vi "AlliGator Build Background Dataset Information String.vi"(8 "error in (no error)":errorcluster, 11 "Bkgd Subtraction":bool) -> (0 "error out":errorcluster, 3 "Background Dataset Description":string)   [LabVIEW 2021, in "AlliGator Files.lvlib"]
doc: "Builds background dataset information string."
uses:
  AlliGator Files.lvlib
  Globals, Variables, Constants/AlliGator Variables List.ctl
  Variant/Variant to Data/Variant to Path.vi
  Variant/Variant to Data/Variant to Boolean.vi
  Variant/Variant to Data/Variant to U32.vi
  Variant/Variant to Data/Variant to DBL.vi
  Variant/Variant to Data/Variant to String.vi
  Globals, Variables, Constants/AlliGator Globals, Variables & Constants.lvlib
  Variant/Variant to Data/Variant to Data.lvlib
panel:
  # "see the AlliGator License on the block diagram (Ctrl+E or Window:Show Block Diagram)"
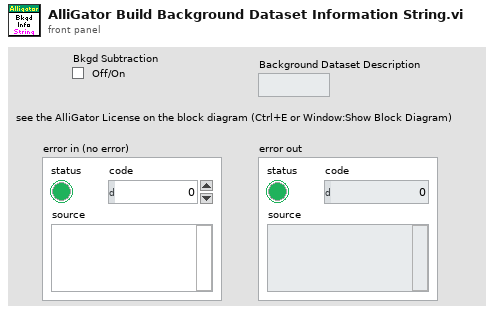
[diagram p1: front panel]
types:
  T1 = typedef "AlliGator Globals, Variables & Constants.lvlib/AlliGator Variables List.ctl" = enum16{"---- GUI ----", "GUI:Initialization Status", "GUI:State Indicators Refnum", "GUI:Original AlliGator Menu Items", "GUI:Current Action Loop State", "GUI:Script in progress", "GUI:Playback", "GUI:Loop Playback", "GUI:Search ROI Used", "GUI:Search ROI", "Decay Graph Max Legend Size", "Intensity Graph Max Legend Size", "Decay Statistics Graph Max Legend Size", "Phasor Graph Max Legend Size", "Phasor Ratio Graph Max Legend Size", "Lifetime Graph Max Legend Size", "---- Files ----", "Files:Export Dataset Frames as Individual Files", "Files:Show Batch Export Help Balloons", "Files:Frames in Dataset", "Files:ptu File Frame Start Indices", "Files:Current Frame in Dataset", "Files:Current Frame Timestamp", "Files:Dataset Loaded", "Files:Dataset Metadata", "Files:Dataset Channel", "Files:Dataset Data Description", "Files:Background Dataset Metadata", "Files:Background Dataset Channel", "Files:Background Dataset Data Description", "Files:Background File Subtraction", "Files:Background File Path", "Files:Background File Pile-up Correction", "Files:Background File Pixel Well Capacity", "Files:Background File Scaling Factor", "Files:Current Dataset Load Settings", "Files:Dataset Path", "Files:ICCD-specific Information", "Files:Macrotime Gate Separation", "------ Python Plugins ------", "Python Plugins:Information", "Python Plugins:Python Session", "Python Plugins:Valid Python Session?", "---- Source Image ----", "Source Image:ROIs", "Source Image:Current ROI", "Source Image:ROI Event Refnum", "X_Source Image Display Range", "X_Source Image Palette Information", "X_Type of Displayed Image", "X_Time Gate Slider", "Source Image:Palette List", "Source Image:Scale", "Source Image:ROI Overlay Color", "Source Image:Overlay to Erase", "Source Image:Is Displayed Image Accumulated", "Source Image:White Light Image Modified", "Source Image:Mask Image Modified", "---- Image Profile Window ----", "Image Profile:Window Event Refnum", "Image Profile:IntensityType", "Image Profile:Intensity Average Type", "Image Profile:Intensity-weighted SDV", "Image Profile:Box Profile Type", "Image Profile:Window Open", "Image Profile:Plotted Fit Parameter", "------ Phasor Graph -------", "Phasor Graph:Show Line", "---- Phasor Plot ---", "Phasor Plot:Parameters Changed", "Phasor Plot:FLI Dataset Modified since last Calculation", "Phasor Harmonics Data", "Selected Phasor Harmonics", "Phasor Harmonic Manager Event Refnum", "Phasor Plot:ROIs", "Phasor Plot:Current ROI", "Phasor Plot:ROI Event Refnum", "Phasor Plot:Image Reference Points", "Phasor Plot:Computed", "Phasor Plot:Palette Information", "Phasor Plot:Palette List", "Phasor Plot:Phasor Ratio Palette Information", "Phasor Plot:Phasor Ratio Palette List", "Phasor Plot:Image Scale", "Phasor Plot:Image Overlay to Erase", "Phasor Plot:Image Elements to Update", "Phasor Plot:Current Calculation Parameters", "Phasor Plot:Current Calibration Options", "Phasor Plot:Reset Cumulated Phasor Plot", "Phasor Plot:Reference 1", "Phasor Plot:Lifetime Reference 1", "Phasor Plot:Reference 1 Frequency", "Phasor Plot:Reference 2", "Phasor Plot:Lifetime Reference 2", "Phasor Plot:Reference 2 Frequency", "---- Decay Analysis ----", "Number of Selected Decays to Fit", "LS Fit Results", "LAR Fit Results", "BS Fit Results", "Last Decay Max - Min", "Best Fit Parameters", "Best Fit Parameter Names", "Actual Size X", "Actual Size Y", "Binning X", "Binning Y", "Actual # Gates", "Dataset Number", "Gates to...", "Gates Skipped", "Gates to keep", "Gate Step", "Gate Separation", "Reversed Gates", "Pile-up Correction", "Pixel Well Capacity", "Background Subtracted", "Background Subtraction Method", "Background Definition Range", "Background File (deprecated)", "Number of Dataset Accumulated", "Array of Accumulated Dataset Paths", "Do Averaged Datasets", "Destination File Path", "Process Plot Target", "Use 1/D as Phasor Frequency", "---- Decay Fit Parameter Map -----", "Decay Fit Parameter Map:Palette Information", "Decay Fit Parameter Map:Palette List", "---- Parameter Map ----", "Parameter Map:Palette Information", "Parameter Map:Palette List", "------- Local Decay Window ---------", "Local Decay Graph Window:Event Refnum", "Local Decay Graph Window:Use normalized IRF for convolution", "----- Miscellaneous ----", "Misc:Skippable Dialog Windows Status"}
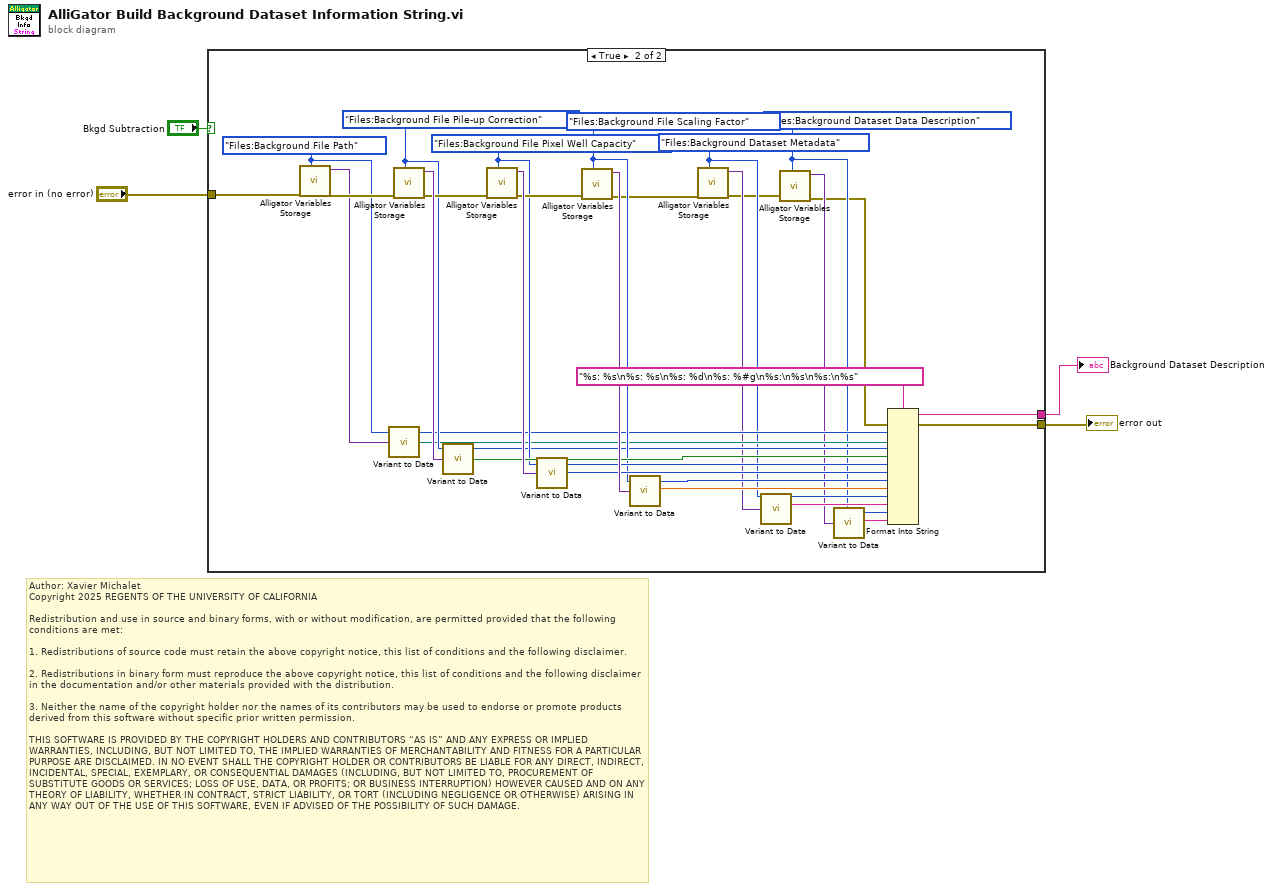
[diagram p0: block diagram]
diagram:
  # "Author: Xavier Michalet\nCopyright 2025 REGENTS OF THE UNIVERSITY OF CALIFORNIA\n\nRedistribution and use in source and binary forms, with or without modification, are permitted provided that the following conditions are met:\n\n1. Redistributions of source code must retain the above copyright notice, this list of conditions and the following disclaimer.\n\n2. Redistributions in binary form must reproduce the above copyright notice, this list of conditions and the following disclaimer in the documentation and/or other materials provided with the distribution.\n\n3. Neither the name of the copyright holder nor the names of its contributors may be used to endorse or promote products derived from this software without specific prior written permission.\n\nTHIS SOFTWARE IS PROVIDED BY THE COPYRIGHT HOLDERS AND CONTRIBUTORS “AS IS” AND ANY EXPRESS OR IMPLIED WARRANTIES, INCLUDING, BUT NOT LIMITED TO, THE IMPLIED WARRANTIES OF MERCHANTABILITY AND FITNESS FOR A PARTICULAR PURPOSE ARE DISCLAIMED. IN NO EVENT SHALL THE COPYRIGHT HOLDER OR CONTRIBUTORS BE LIABLE FOR ANY DIRECT, INDIRECT, INCIDENTAL, SPECIAL, EXEMPLARY, OR CONSEQUENTIAL DAMAGES (INCLUDING, BUT NOT LIMITED TO, PROCUREMENT OF SUBSTITUTE GOODS OR SERVICES; LOSS OF USE, DATA, OR PROFITS; OR BUSINESS INTERRUPTION) HOWEVER CAUSED AND ON ANY THEORY OF LIABILITY, WHETHER IN CONTRACT, STRICT LIABILITY, OR TORT (INCLUDING NEGLIGENCE OR OTHERWISE) ARISING IN ANY WAY OUT OF THE USE OF THIS SOFTWARE, EVEN IF ADVISED OF THE POSSIBILITY OF SUCH DAMAGE."
  n1 = case shown="True" "Bkgd Subtraction" {
    tunnel: [_ w33] -> w4
    tunnel: "error in (no error)" -> [w5 w21]
    tunnel: [w5 w7] -> w2
    frame False {
    }
    frame True {
      w11 = AlliGator_Variables_List."Files:Background Dataset Data Description" ("Alligator Variable")
      w14 = AlliGator_Variables_List."Files:Background Dataset Metadata" ("Alligator Variable")
      w17 = AlliGator_Variables_List."Files:Background File Path" ("Alligator Variable")
      w24 = AlliGator_Variables_List."Files:Background File Scaling Factor" ("Alligator Variable")
      w26 = AlliGator_Variables_List."Files:Background File Pixel Well Capacity" ("Alligator Variable")
      w22 = AlliGator_Variables_List."Files:Background File Pile-up Correction" ("Alligator Variable")
      n2 = call "Alligator Variables Storage.vi"("AlliGator Variable"=w17, "Error In"=w21) -> ("Error Out"=w20:errorcluster, "Data out"=w19:variant)  [unwired: 7 in, 1 out]
      n3 = call-poly "Variant to Data.vi"("Variant"=w19) -> ("Path"=w18:path)  [unwired: 8 in]
      n4 = call "Alligator Variables Storage.vi"("AlliGator Variable"=w22, "Error In"=w20) -> ("Error Out"=w31:errorcluster, "Data out"=w32:variant)  [unwired: 7 in, 1 out]
      n5 = call-poly "Variant to Data.vi"("Variant"=w32) -> ("Value"=w27:bool)  [unwired: 8 in]
      n6 = call "Alligator Variables Storage.vi"("AlliGator Variable"=w26, "Error In"=w31) -> ("Error Out"=w29:errorcluster, "Data out"=w30:variant)  [unwired: 7 in, 1 out]
      n7 = call-poly "Variant to Data.vi"("Variant"=w30) -> ("Value"=w25:u32)  [unwired: 8 in]
      n8 = call "Alligator Variables Storage.vi"("AlliGator Variable"=w24, "Error In"=w29) -> ("Error Out"=w16:errorcluster, "Data out"=w28:variant)  [unwired: 7 in, 1 out]
      n9 = call-poly "Variant to Data.vi"("Variant"=w28) -> ("Value"=w23:dbl)  [unwired: 8 in]
      n10 = call "Alligator Variables Storage.vi"("AlliGator Variable"=w14, "Error In"=w16) -> ("Error Out"=w12:errorcluster, "Data out"=w15:variant)  [unwired: 7 in, 1 out]
      n11 = call-poly "Variant to Data.vi"("Variant"=w15) -> ("String"=w13:string)  [unwired: 8 in]
      n12 = call "Alligator Variables Storage.vi"("AlliGator Variable"=w11, "Error In"=w12) -> ("Error Out"=w8:errorcluster, "Data out"=w10:variant)  [unwired: 7 in, 1 out]
      n13 = call-poly "Variant to Data.vi"("Variant"=w10) -> ("String"=w9:string)  [unwired: 8 in]
      n14 = Format Into String(format string="%s: %s\n%s: %s\n%s: %d\n%s: %#g\n%s:\n%s\n%s:\n%s", error in=w8, w17, w18, w22, w27, w26, w25, w24, w23, w14, w13, w11, w9) -> (resulting string=w33:string, error out=w7:errorcluster)  [unwired: 1 in]
    }
  }
  "Background Dataset Description" <- w4
  "error out" <- w2
